vi "S2C_FORNAX_Poly_DftInstrumentCommand.vi"(8 "Error In":errorcluster, 10 "DftInstrumentCommand":T3={"Partition"="Default", "Message"="DftInstrumentCommand", "M_EnergyChannelId"=0, "M_DftInstrumentCommand"=0, "M_IntValue"=0, "M_FloatValue"=0.0, "M_StringValue"=""} {"M_DftInstrumentCommand" items=["DFT_INSTRUMENT_COMMAND_NONE", "DFT_INSTRUMENT_COMMAND_SCAN", "DFT_INSTRUMENT_COMMAND_SCAN_BARCODE", "DFT_INSTRUMENT_COMMAND_SCAN_RFID", "DFT_INSTRUMENT_COMMAND_USE_INSTRUMENT_TYPE", "DFT_INSTRUMENT_COMMAND_USE_ACCESSORY_ID", "DFT_INSTRUMENT_COMMAND_WRITE_RFID_USAGE_INFO", "DFT_INSTRUMENT_COMMAND_SKIP_RFID_CHECKS", "DFT_INSTRUMENT_COMMAND_SKIP_RFID_TIMESTAMP_WRITE", "DFT_INSTRUMENT_COMMAND_SKIP_RFID_SIGNATURE_WRITE", "DFT_INSTRUMENT_COMMAND_FORCE_RFID_SIGNATURE_WRITE", "DFT_INSTRUMENT_COMMAND_CYCLE_INSERTIONS", "DFT_INSTRUMENT_COMMAND_INSERTION_DEBOUNCING"]; "M_EnergyChannelId" items=["EC_MONO_1"=0, "EC_BIPOLAR"=1, "EC_MONO_2"=2, "EC_ADVANCED"=3, "EC_ADVANCED_ECUT"=4, "EC_ADVANCED_DCUT"=5, "EC_SHARED_COAG"=6, "EC_INTERNAL_BIP_CAL"=7, "EC_NOT_USED"=-1]}, 11 "Settings":T4={"Driver"="Fornax", "Command"="DftInstrumentCommand", "Return"="ErrorStatus", "Parameters"="", "Timeout"=10.0}) -> (0 "Error Out":errorcluster, 3 "Response":string)   [LabVIEW 2015]
uses:
  Typedefs/EnergyChannelId.ctl
  Typedefs/DftInstrumentCommand.ctl
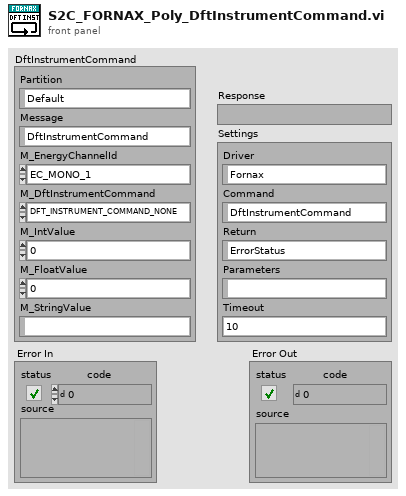
[diagram p1: front panel]
types:
  T1 = typedef "EnergyChannelId.ctl" = i16
  T2 = typedef "DftInstrumentCommand.ctl" = i16
  T3 = cluster{"Partition":string, "Message":string, "M_EnergyChannelId":T1, "M_DftInstrumentCommand":T2, "M_IntValue":i32, "M_FloatValue":dbl, "M_StringValue":string}
  T4 = cluster{"Driver":string, "Command":string, "Return":string, "Parameters":string, "Timeout":dbl}
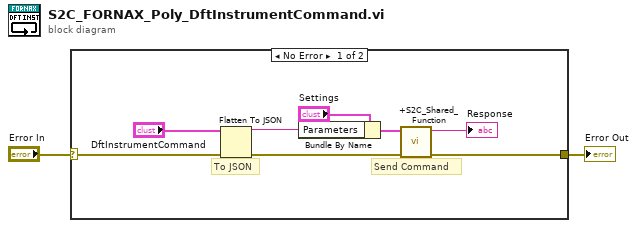
[diagram p0: block diagram]
diagram:
  n1 = case shown="No Error" "Error In" {
    selector: "Error In" -> [w6 w11]
    tunnel: [w5 w11] -> w1
    frame No Error {
      # "To JSON"
      # "Send Command"
      n2 = Flatten To JSON(anything="DftInstrumentCommand", error in (no error)=w6) -> (JSON string=w7:string, 11:w9:errorcluster)  [unwired: 1 in]
      n3 = Bundle By Name(cluster="Settings", "Parameters"=w7) -> (w10:T4)
      n4 = call "+S2C_Shared_Function.vi"("Error In"=w9, "Settings"=w10) -> ("Error Out"=w5:errorcluster, "Response"=→"Response":string)  [unwired: 8 in]
    }
    frame Error {
    }
  }
  "Error Out" <- w1
